vi "Interpret_Read Registers.vi"(8 "error in (no error)":errorcluster, 11 "MB_PDU_resp in":T1={"Function Code"=1, "Data"=[], "RTU_DataBytes"=0}) -> (0 "error out":errorcluster, 2 "Registers":u16[](array[numeric]))   [LabVIEW 2023, in "MB Master.lvlib"]
doc: "Extracts the data of a PDU request/response pair based on the function code of the response.\n\nReturns an array of booleans for coils and discrete inputs.\nReturns an array of unsigned 16-bit integers for input and holding registers."
uses:
  <vilib>/Plasmionique/MB Master/MB Master.lvlib
  <vilib>/Plasmionique/MB Master/MB_PDU/MB_PDU_Cluster.ctl
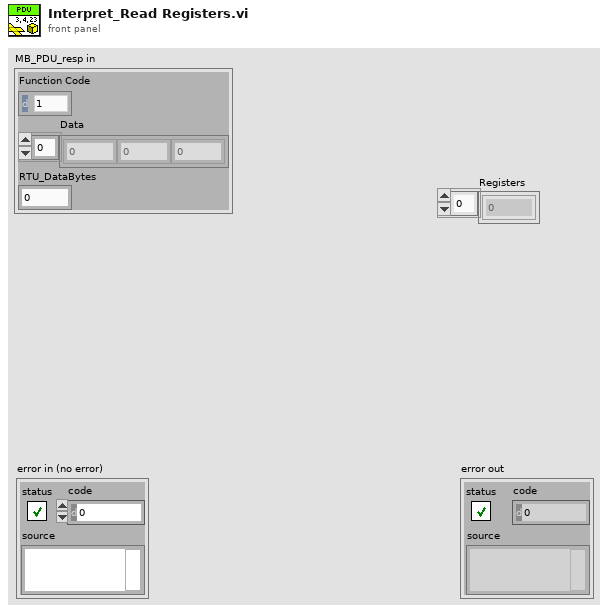
[diagram p1: front panel]
types:
  T1 = typedef "MB Master.lvlib/MB_PDU_Cluster.ctl" = cluster{"Function Code":u8, "Data":u8[], "RTU_DataBytes":i32}
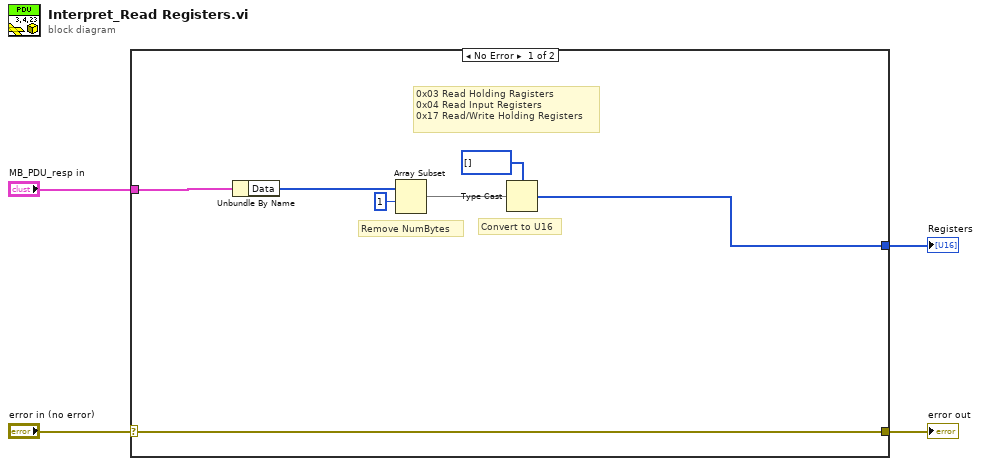
[diagram p0: block diagram]
diagram:
  n1 = case shown="No Error" "error in (no error)" {
    selector: "error in (no error)" -> [w11 w12]
    tunnel: [w11 w12] -> w3
    tunnel: "MB_PDU_resp in" -> [w10 _]
    tunnel: [w8 _] -> w1
    frame No Error {
      # "Convert to U16"
      # "Remove NumBytes"
      # "0x03 Read Holding Ragisters\n0x04 Read Input Registers\n0x17 Read/Write Holding Registers"
      n2 = Unbundle By Name(w10) -> ("Data"=w9:u8[])
      n3 = Array Subset(array=w9, index=1) -> (w6:u8[])  [unwired: 1 in]
      n4 = Type Cast(type=u16[] [], x=w6) -> (*(type *) &x=w8:u16[])
    }
    frame Error {
    }
  }
  "error out" <- w3
  "Registers" <- w1
